vi "upscale_array.vi"(10 "Upsample Factor":i32, 11 "Small Array":u8[][](array[numeric])) -> (2 "Actual Upsample Factor":i32, 3 "Big Array":u8[][](array[numeric]), 5 "Resamples":i32[](array[numeric]))   [LabVIEW 2020]
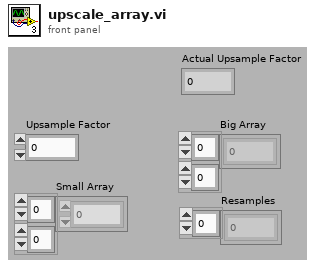
[diagram p1: front panel]
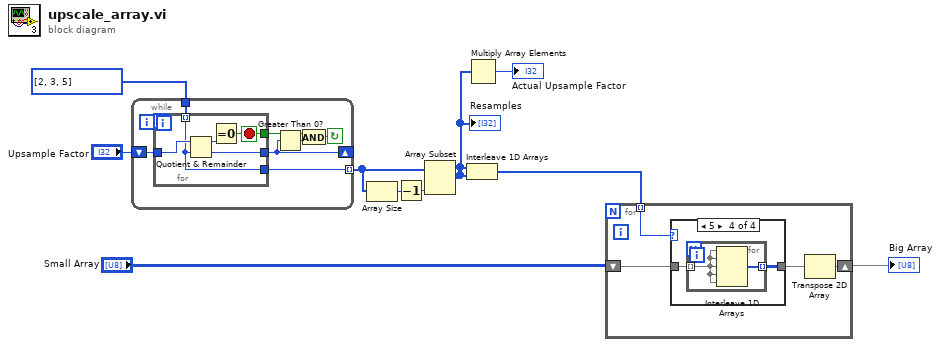
[diagram p0: block diagram]
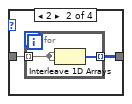
[diagram p3: hidden frame]
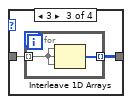
[diagram p4: hidden frame]
diagram:
  n1 = while {
    tunnel: i32[] [2, 3, 5] -> [w16]
    shift-right: [w11] -> _
    shift-left: "Upsample Factor" -> [w17]
    tunnel: [w14] -> w5 mode=indexing
    stop <- w13 continue-if-true
    n2 = for {
      tunnel: w17 -> [w22]
      tunnel: w16 -> [w18] mode=indexing
      tunnel: [w20] -> w15
      tunnel: [w19] -> w11
      tunnel: [w18] -> w14
      stop <- w20 stop-if-true
      n3 = Quotient & Remainder(x=w22, y=w18) -> (x-y*floor(x/y)=w21:i32, floor(x/y)=w19:i32)
      n4 = Equal To 0?(x=w21) -> (x = 0?=w20:bool)
    }
    n5 = Greater Than 0?(x=w11) -> (x > 0?=w12:bool)
    n6 = And(x=w15, y=w12) -> (x .and. y?=w13:bool)
  }
  n7 = Array Size(array=w5) -> (size(s)=w6:i32)
  n8 = Decrement(x=w6) -> (x-1=w4:i32)
  n9 = Array Subset(array=w5, length=w4) -> (w2:i32[])  [unwired: 1 in]
  "Resamples" <- w2
  n10 = Interleave 1D Arrays(w2, w2) -> (w3:i32[])
  n11 = Multiply Array Elements(1:w2) -> (0:→"Actual Upsample Factor":i32)
  n12 = for {
    shift-right: [w24] -> w10
    shift-left: "Small Array" -> [w26]
    tunnel: w3 -> [w23] mode=indexing
    n13 = case shown="5" w23 {
      tunnel: w26 -> [w27 w29 w33 w37]
      tunnel: [w27 w28 w32 w36] -> w25
      frame 0, Default {
      }
      frame 2 {
        n14 = for {
          tunnel: w29 -> [w30] mode=indexing
          tunnel: [w31] -> w28 mode=indexing
          n15 = Interleave 1D Arrays(w30, w30) -> (w31:u8[])
        }
      }
      frame 3 {
        n16 = for {
          tunnel: w33 -> [w34] mode=indexing
          tunnel: [w35] -> w32 mode=indexing
          n17 = Interleave 1D Arrays(w34, w34, w34) -> (w35:u8[])
        }
      }
      frame 5 {
        n18 = for {
          tunnel: w37 -> [w38] mode=indexing
          tunnel: [w39] -> w36 mode=indexing
          n19 = Interleave 1D Arrays(w38, w38, w38, w38, w38) -> (w39:u8[])
        }
      }
    }
    n20 = Transpose 2D Array(2D array=w25) -> (transposed array=w24:u8[][])
  }
  "Big Array" <- w10
